vi "gantry移動定位_六邊形(內切圓).vi"() -> ()   [LabVIEW 2016]
uses:
  Classes/Controller/Motion/A3200 Folder/A3200.lvclass
panel:
  out "點座標":dbl[][](array[numeric])
  in  "內切圓半徑":dbl=100.0
  in  "中心點座標":dbl[](array[numeric])
  out "Final Position":dbl[](array[numeric])
  out "Initial position":dbl[](array[numeric])
  in  "Speed (mm/s)":dbl=40.0
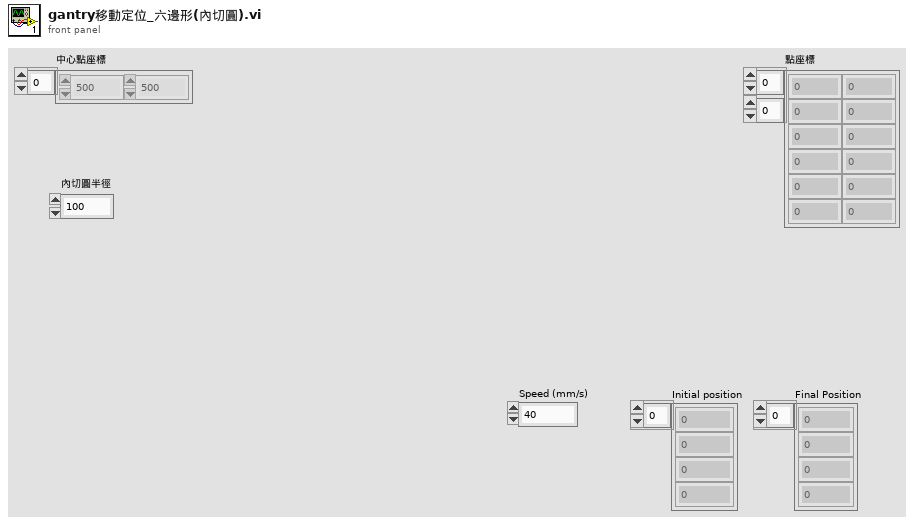
[diagram p1: front panel]
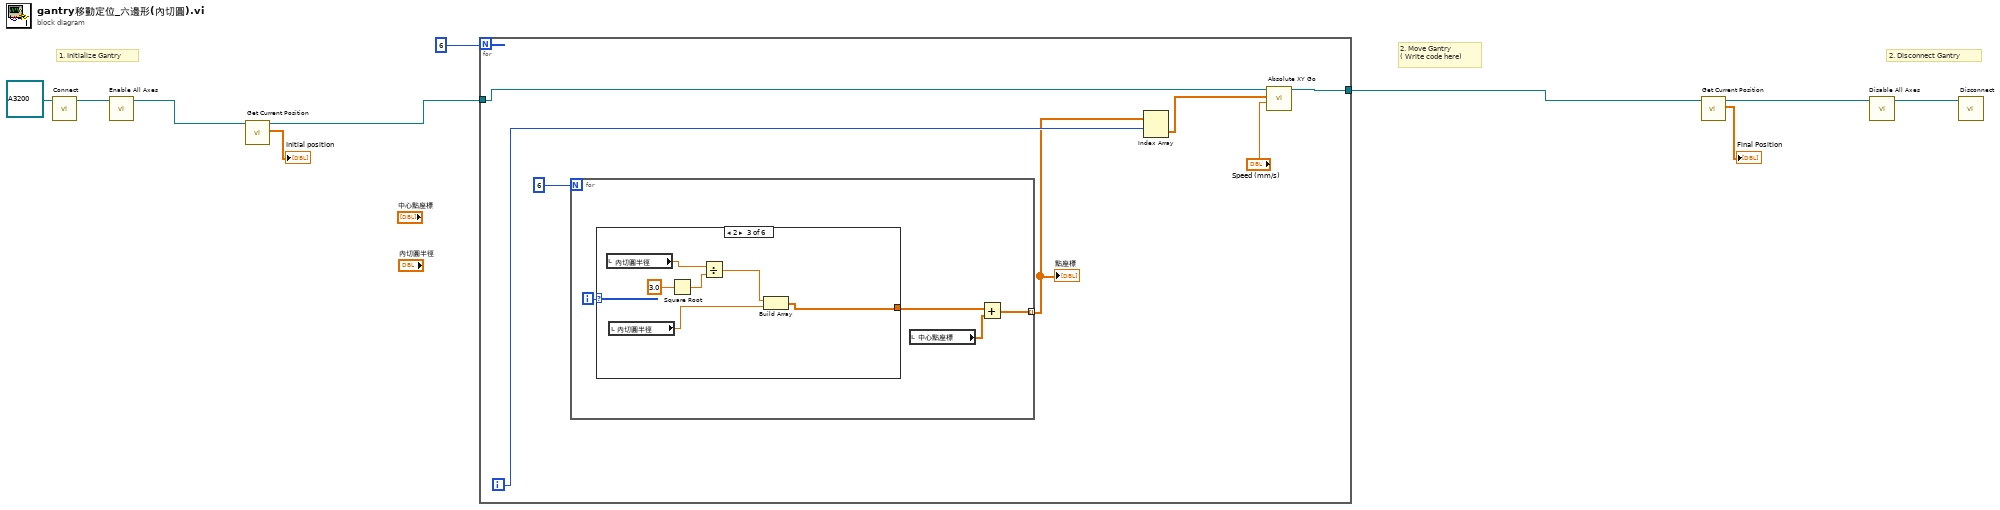
[diagram p0: block diagram]
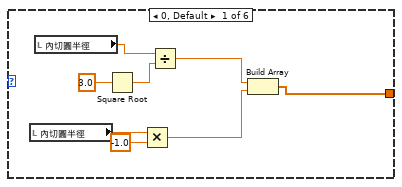
[diagram p2: hidden frame]
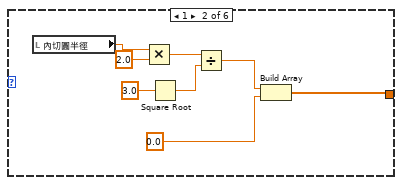
[diagram p3: hidden frame]
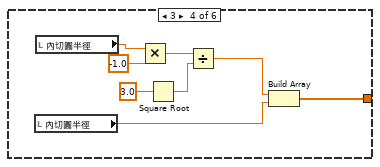
[diagram p4: hidden frame]
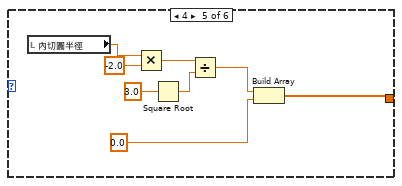
[diagram p5: hidden frame]
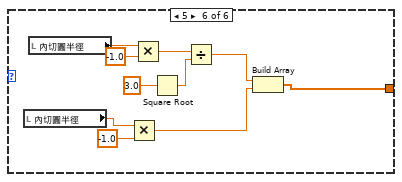
[diagram p6: hidden frame]
diagram:
  # "1. Initialize Gantry"
  # "2. Disconnect Gantry"
  # "2. Move Gantry \n( Write code here)"
  n1 = call-dynamic "Connect.vi"("Gantry in"=refnum<class "A3200.lvclass"> refnum ("A3200.lvclass")) -> ("Gantry out"=w5:refnum<class "A3200.lvclass">)  [unwired: 9 in, 1 out]
  n2 = call-dynamic "Enable All Axes.vi"("A3200 in"=w5) -> ("A3200 out"=w4:refnum<class "A3200.lvclass">)  [unwired: 9 in, 1 out]
  n3 = call-dynamic "Get Current Position.vi"("Gantry in"=w4) -> ("XYZTheta Out"=→"Initial position":dbl[], "Gantry out"=w3:refnum<class "A3200.lvclass">)  [unwired: 8 in, 1 out]
  n4 = for {
    N: 6 -> [_]
    tunnel: w3 -> [w15]
    tunnel: [w14] -> w2
    i -> [w17]
    n5 = for {
      N: 6 -> [_]
      tunnel: [w18] -> w12 mode=indexing
      i -> [w21]
      n6 = case shown="2" w21 {
        tunnel: [w22 w30 w38 w44 w52 w60] -> w20
        frame 0, Default {
          n7 = local read "內切圓半徑"() -> (w26:dbl)
          n8 = local read "內切圓半徑"() -> (w29:dbl)
          n9 = Square Root(x=3.0) -> (sqrt(x)=w27:dbl)
          n10 = Multiply(x=w26, y=-1.0) -> (x*y=w23:dbl)
          n11 = Divide(x=w29, y=w27) -> (x/y=w24:dbl)
          n12 = Build Array(w24, w23) -> (w22:dbl[])
        }
        frame 1 {
          n13 = local read "內切圓半徑"() -> (w37:dbl)
          n14 = Multiply(x=w37, y=2.0) -> (x*y=w35:dbl)
          n15 = Square Root(x=3.0) -> (sqrt(x)=w33:dbl)
          n16 = Divide(x=w35, y=w33) -> (x/y=w32:dbl)
          n17 = Build Array(w32, 0.0) -> (w30:dbl[])
        }
        frame 2 {
          n18 = local read "內切圓半徑"() -> (w43:dbl)
          n19 = local read "內切圓半徑"() -> (w39:dbl)
          n20 = Square Root(x=3.0) -> (sqrt(x)=w41:dbl)
          n21 = Divide(x=w43, y=w41) -> (x/y=w40:dbl)
          n22 = Build Array(w40, w39) -> (w38:dbl[])
        }
        frame 3 {
          n23 = local read "內切圓半徑"() -> (w45:dbl)
          n24 = local read "內切圓半徑"() -> (w51:dbl)
          n25 = Multiply(x=w51, y=-1.0) -> (x*y=w49:dbl)
          n26 = Square Root(x=3.0) -> (sqrt(x)=w47:dbl)
          n27 = Divide(x=w49, y=w47) -> (x/y=w46:dbl)
          n28 = Build Array(w46, w45) -> (w44:dbl[])
        }
        frame 4 {
          n29 = local read "內切圓半徑"() -> (w59:dbl)
          n30 = Multiply(x=w59, y=-2.0) -> (x*y=w57:dbl)
          n31 = Square Root(x=3.0) -> (sqrt(x)=w55:dbl)
          n32 = Divide(x=w57, y=w55) -> (x/y=w54:dbl)
          n33 = Build Array(w54, 0.0) -> (w52:dbl[])
        }
        frame 5 {
          n34 = local read "內切圓半徑"() -> (w64:dbl)
          n35 = local read "內切圓半徑"() -> (w69:dbl)
          n36 = Multiply(x=w64, y=-1.0) -> (x*y=w61:dbl)
          n37 = Multiply(x=w69, y=-1.0) -> (x*y=w67:dbl)
          n38 = Square Root(x=3.0) -> (sqrt(x)=w66:dbl)
          n39 = Divide(x=w67, y=w66) -> (x/y=w62:dbl)
          n40 = Build Array(w62, w61) -> (w60:dbl[])
        }
      }
      n41 = local read "中心點座標"() -> (w19:dbl[])
      n42 = Add(x=w20, y=w19) -> (x+y=w18:dbl[])
    }
    "點座標" <- w12
    n43 = Index Array(array=w12, index (row)=w17) -> (element=w11:dbl[])  [unwired: 1 in]
    n44 = call-dynamic "Absolute XY Go.vi"("Speed"="Speed (mm/s)", "XY"=w11, "Gantry in"=w15) -> ("Gantry out"=w14:refnum<class "A3200.lvclass">)  [unwired: 7 in, 1 out]
  }
  n45 = call-dynamic "Get Current Position.vi"("Gantry in"=w2) -> ("XYZTheta Out"=→"Final Position":dbl[], "Gantry out"=w8:refnum<class "A3200.lvclass">)  [unwired: 8 in, 1 out]
  n46 = call-dynamic "Disable All Axes.vi"("Gantry in"=w8) -> ("Gantry out"=w9:refnum<class "A3200.lvclass">)  [unwired: 9 in, 1 out]
  n47 = call-dynamic "Disconnect.vi"("Gantry in"=w9) -> ()  [unwired: 9 in, 1 out]
